vi "Escape String.vi"(5 "Escape string? [T]":bool=TRUE, 7 "Essential only? [F]":bool, 8 "error in (no error)":errorcluster, 10 "String":string, 11 "Registry Object":refnum<class "Carya Config.lvclass">) -> (0 "error out":errorcluster, 2 "Escaped string":string, 3 "Registry Object":refnum<class "Carya Config.lvclass">)   [LabVIEW 2013, in "Carya Config.lvclass"]
doc: "Copyright 2018, Carya Automatisering, Wiebe Walstra."
uses:
  Carya Config.lvclass
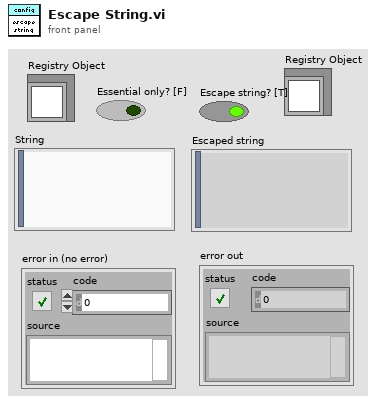
[diagram p1: front panel]
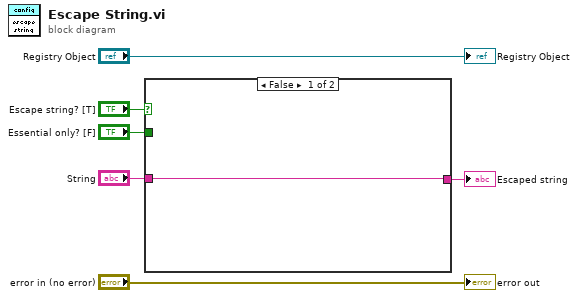
[diagram p0: block diagram]
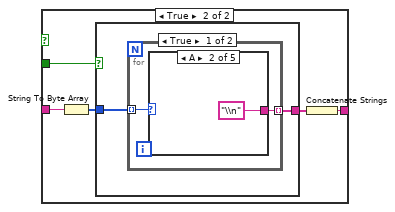
[diagram p2: hidden frame]
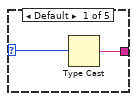
[diagram p3: hidden frame]
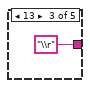
[diagram p4: hidden frame]
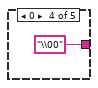
[diagram p5: hidden frame]
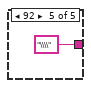
[diagram p6: hidden frame]
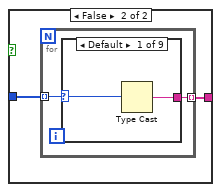
[diagram p7: hidden frame]
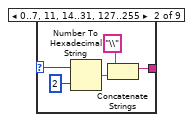
[diagram p8: hidden frame]
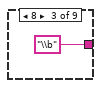
[diagram p9: hidden frame]
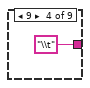
[diagram p10: hidden frame]
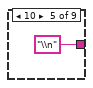
[diagram p11: hidden frame]
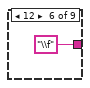
[diagram p12: hidden frame]
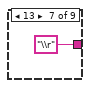
[diagram p13: hidden frame]
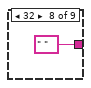
[diagram p14: hidden frame]
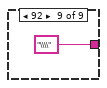
[diagram p15: hidden frame]
diagram:
  n1 = case shown="False" "Escape string? [T]" {
    tunnel: [w7 w12] -> w5
    tunnel: "String" -> [w7 w11]
    tunnel: "Essential only? [F]" -> [_ w8]
    frame False {
    }
    frame True {
      n2 = String To Byte Array(string=w11) -> (unsigned byte array=w10:u8[])
      n3 = case shown="True" w8 {
        tunnel: w10 -> [w14 w24]
        tunnel: [w13 w23] -> w9
        frame True {
          n4 = for {
            tunnel: w14 -> [w15] mode=indexing
            tunnel: [w16] -> w13 mode=indexing
            n5 = case shown="A" w15 {
              selector: w15 -> [w17 _ _ _ _]
              tunnel: [w18 "\\n" "\\r" "\\00" "\\\\"] -> w16
              frame Default {
                n6 = Type Cast(x=w17) -> (*(type *) &x=w18:string)  [unwired: 1 in]
              }
              frame 10 {
              }
              frame 13 {
              }
              frame 0 {
              }
              frame 92 {
              }
            }
          }
        }
        frame False {
          n7 = for {
            tunnel: w24 -> [w25] mode=indexing
            tunnel: [w26] -> w23 mode=indexing
            n8 = case shown="Default" w25 {
              selector: w25 -> [w27 w29 _ _ _ _ _ _ _]
              tunnel: [w28 w31 "\\b" "\\t" "\\n" "\\f" "\\r" " " "\\\\"] -> w26
              frame Default {
                n9 = Type Cast(x=w27) -> (*(type *) &x=w28:string)  [unwired: 1 in]
              }
              frame 0..7, 11, 14..31, 127..255 {
                n10 = Number To Hexadecimal String(1:i16 2 ("width (-)"), 2:w29) -> (0:w32:string)
                n11 = Concatenate Strings("\\" ("string"), w32) -> (w31:string)
              }
              frame 8 {
              }
              frame 9 {
              }
              frame 10 {
              }
              frame 12 {
              }
              frame 13 {
              }
              frame 32 {
              }
              frame 92 {
              }
            }
          }
        }
      }
      n12 = Concatenate Strings(w9) -> (w12:string)
    }
  }
  "Escaped string" <- w5
  "Registry Object" <- "Registry Object"
  "error out" <- "error in (no error)"
